vi "Pasco Auton Drive Shoot.vi"(0 "Desired Heading":dbl, 1 "Actual Heading":dbl, 2 "time/distance":dbl, 3 "Power":dbl, 4 "Array":i32, 5 "Encoder total":dbl, 6 "Time":i32, 7 "Encoder Return":dbl) -> (14 "Left Drive":dbl, 15 "Right Drive":dbl, 16 "Array Out":i32, 17 "Encoder total":dbl)   [LabVIEW 2011]
uses:
  <vilib>/addons/control/pid/pid.llb/PID (DBL).vi
  <vilib>/addons/control/pid/NI_PID_pid.lvlib
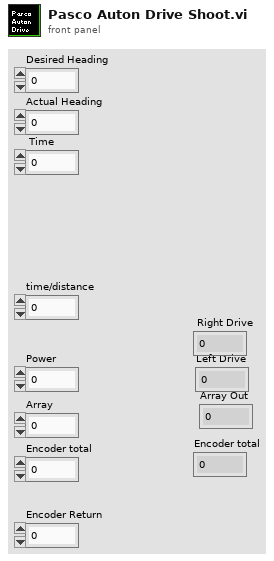
[diagram p1: front panel]
types:
  T1 = cluster{"proportional gain (Kc)":dbl, "integral time (Ti, min)":dbl, "derivative time (Td, min)":dbl}
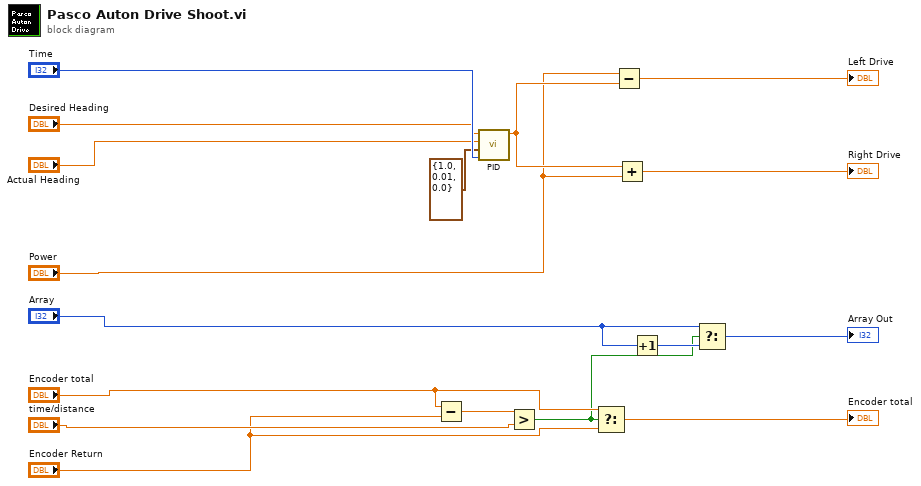
[diagram p0: block diagram]
diagram:
  n1 = Subtract(x="Encoder total", y="Encoder Return") -> (x-y=w17:dbl)
  n2 = call-poly <vilib>:"PID.vi"("dt (s)"="Time", "PID gains"=T1 {"proportional gain (Kc)"=1.0, "integral time (Ti, min)"=0.01, "derivative time (Td, min)"=0.0}, "process variable"="Actual Heading", "setpoint"="Desired Heading") -> ("output"=w16:dbl)  [unwired: 6 in, 1 out]
  n3 = Greater?(x=w17, y="time/distance") -> (0:w6:bool)
  n4 = Select(t="Encoder total", s=w6, f="Encoder Return") -> (s? t:f=→"Encoder total":dbl)
  n5 = Subtract(x="Power", y=w16) -> (x-y=→"Left Drive":dbl)
  n6 = Add(x=w16, y="Power") -> (x+y=→"Right Drive":dbl)
  n7 = Increment(x="Array") -> (x+1=w7:i32)
  n8 = Select(t="Array", s=w6, f=w7) -> (s? t:f=→"Array Out":i32)
